vi "System Explorer - Copy Templates for System Explorer.vi"(7 "CD Name":string, 8 "error in (no error)":errorcluster, 10 "CD Template":refnum<class "NIVS_CD Template.lvclass">, 11 "System Explorer folder":path) -> (0 "error out":errorcluster)   [LabVIEW 2020, in "NIVS_Consolidated_CDW_MetaDataObj.lvclass"]
doc: "Copy the templates for the System Explorer library into the System Explorer folder and disconnect the templates from the owning library."
uses:
  NIVS_Consolidated_CDW_MetaDataObj.lvclass
  Template Classes/NIVS_CD Template/NIVS_CD Template.lvclass
  CD System Explorer lvlib.ctl
  Common.ctl
  CD Shared lvlib.ctl
  CD System Explorer lvlib.vi
  Common.vi
  CD Shared lvlib.vi
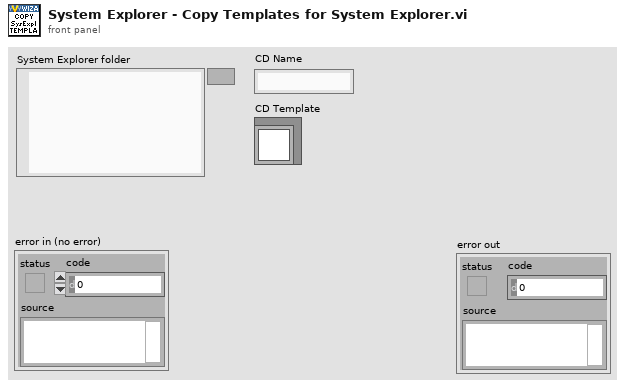
[diagram p1: front panel]
types:
  T1 = typedef "NIVS_Consolidated_CDW_MetaDataObj.lvclass/CD Shared lvlib.ctl" = enum16{"LibraryFileName", "LibraryFolderName", "ConstantsVI.VIPathAndName", "Shared.FolderName", "Shared.Types.FolderName", "Shared.Constants.VIName", "Shared.Constants.VITemplateName", "Shared.Constants.VITemplatePathAndName", "Shared.CompiledSettings.RelativePath", "Shared.Constants.RelativePath", "Shared.CompiledSettings.Name", "Shared.CompiledSettings.Name.NoExtension", "Shared.CompiledSettings.ClusterName"}
  T2 = typedef "NIVS_Consolidated_CDW_MetaDataObj.lvclass/CD System Explorer lvlib.ctl" = enum16{"LibraryFileName", "LibraryFolderName", "System Explorer.FolderName", "System Explorer.Dynamically Called.FolderName", "System Explorer.Dynamically Called.Extra Pages.FolderName", "System Explorer.Dynamically Called.Extra Pages.TemplatePathAndName", "System Explorer.Dynamically Called.Main Page.VIName", "System Explorer.Dynamically Called.Main Page.TemplatePathAndName", "System Explorer.Dynamically Called.Initialization VI.VIName", "System Explorer.Dynamically Called.Initialization VI.TemplatePathAndName", "System Explorer.SubVI.FolderName", "System Explorer.Types.FolderName", "System Explorer.ActionVIOnCompile.VIName", "System Explorer.ExportConfigRTM.VIName", "System Explorer.PPL.ExportConfigRTM.VIName", "System Explorer.LoadHelpFile.VIName", "System Explorer.PPL.LoadHelpFile.VIName", "System Explorer.SetRTDriverVIsFilePaths.VIName", "System Explorer.ClearRTDriverVIs.VIName"}
  T3 = typedef "NIVS_Consolidated_CDW_MetaDataObj.lvclass/Common.ctl" = enum16{"ProjectName", "TemplatesFolderName", "PPLTemplatesFolderName", "ProjectTemplatePathAndName", "ProjectPPLTemplatePathAndName", "TimingAndSyncFolderName", "CustomDeviceFolderName", "PathToTemplates", "PathToPPLTemplates", "PathToExplorerPPLTemplates", "PathToEnginePPLTemplates", "PathToConfigurationFile", "ProjectConfigurationName"}
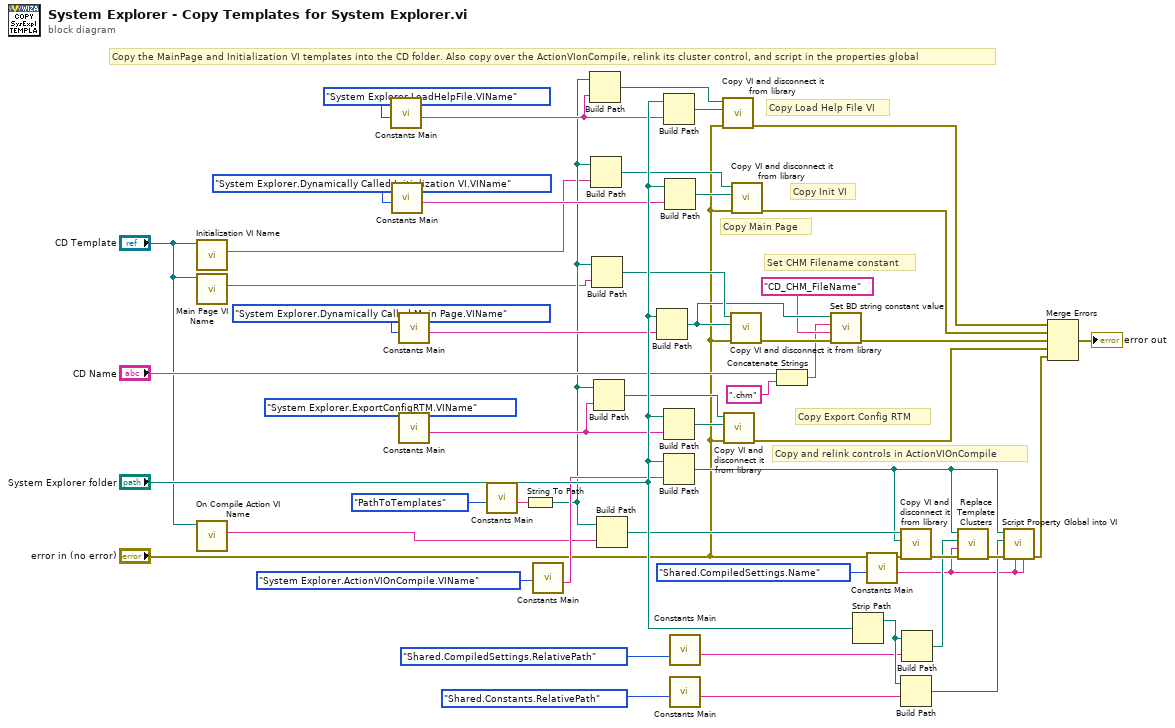
[diagram p0: block diagram]
diagram:
  # "Copy Load Help File VI"
  # "Copy the MainPage and Initialization VI templates into the CD folder. Also copy over the ActionVIonCompile, relink its cluster control, and script in the properties global"
  # "Set CHM Filename constant"
  # "Copy Export Config RTM"
  # "Copy and relink controls in ActionVIOnCompile"
  # "Copy Main Page"
  # "Copy Init VI"
  n1 = call-dynamic "Initialization VI Name.vi"("CD Template in"="CD Template") -> ("Initialization VI Name"=w6:string)  [unwired: 10 in]
  n2 = call-dynamic "Main Page VI Name.vi"("CD Template in"="CD Template") -> ("Main Page VI Name"=w5:string)  [unwired: 10 in]
  n3 = call-dynamic "On Compile Action VI Name.vi"("CD Template in"="CD Template") -> ("On Compile Action VI Name"=w4:string)  [unwired: 10 in]
  n4 = call-poly "Constants Main.vi"("Action"=CD_System_Explorer_lvlib."System Explorer.LoadHelpFile.VIName") -> ("Output"=w13:string)  [unwired: 10 in]
  n5 = call-poly "Constants Main.vi"("Action"=CD_System_Explorer_lvlib."System Explorer.Dynamically Called.Initialization VI.VIName") -> ("Output"=w39:string)  [unwired: 10 in]
  n6 = call-poly "Constants Main.vi"("Action"=CD_System_Explorer_lvlib."System Explorer.Dynamically Called.Main Page.VIName") -> ("Output"=w38:string)  [unwired: 10 in]
  n7 = call-poly "Constants Main.vi"("Action"=CD_System_Explorer_lvlib."System Explorer.ExportConfigRTM.VIName") -> ("Output"=w23:string)  [unwired: 10 in]
  n8 = call-poly "Constants Main.vi"("Action"=Common."PathToTemplates") -> ("Output"=w44:string)  [unwired: 10 in]
  n9 = String To Path(string=w44) -> (path=w9:path)
  n10 = call-poly "Constants Main.vi"("Action"=CD_System_Explorer_lvlib."System Explorer.ActionVIOnCompile.VIName") -> ("Output"=w31:string)  [unwired: 10 in]
  n11 = Build Path(base path=w9, name or relative path=w13) -> (appended path=w12:path)
  n12 = Build Path(base path=w9, name or relative path=w6) -> (appended path=w40:path)
  n13 = Build Path(base path=w9, name or relative path=w5) -> (appended path=w41:path)
  n14 = Build Path(base path=w9, name or relative path=w23) -> (appended path=w26:path)
  n15 = Build Path(base path=w9, name or relative path=w4) -> (appended path=w43:path)
  n16 = Build Path(base path="System Explorer folder", name or relative path=w38) -> (appended path=w19:path)
  n17 = Build Path(base path="System Explorer folder", name or relative path=w13) -> (appended path=w11:path)
  n18 = Build Path(base path="System Explorer folder", name or relative path=w23) -> (appended path=w25:path)
  n19 = Build Path(base path="System Explorer folder", name or relative path=w31) -> (appended path=w36:path)
  n20 = Build Path(base path="System Explorer folder", name or relative path=w39) -> (appended path=w47:path)
  n21 = call-poly "Constants Main.vi"("Action"=CD_Shared_lvlib."Shared.CompiledSettings.RelativePath") -> ("Output"=w1:string)  [unwired: 10 in]
  n22 = call-poly "Constants Main.vi"("Action"=CD_Shared_lvlib."Shared.Constants.RelativePath") -> ("Output"=w29:string)  [unwired: 10 in]
  n23 = call "Copy VI and disconnect it from library.vi"("error in (no error)"="error in (no error)", "VI Target Path"=w11, "VI Source Path"=w12) -> ("error out"=w8:errorcluster)  [unwired: 8 in]
  n24 = call "Copy VI and disconnect it from library.vi"("error in (no error)"="error in (no error)", "VI Target Path"=w25, "VI Source Path"=w26) -> ("error out"=w21:errorcluster)  [unwired: 8 in]
  n25 = call "Copy VI and disconnect it from library.vi"("error in (no error)"="error in (no error)", "VI Target Path"=w19, "VI Source Path"=w41) -> ("error out"=w20:errorcluster)  [unwired: 8 in]
  n26 = call "Copy VI and disconnect it from library.vi"("error in (no error)"="error in (no error)", "VI Target Path"=w47, "VI Source Path"=w40) -> ("error out"=w46:errorcluster)  [unwired: 8 in]
  n27 = Concatenate Strings("CD Name", ".chm" ("string")) -> (w15:string)
  n28 = call "Set BD string constant value.vi"("error in (no error)"=w20, "Name of string constant"="CD_CHM_FileName", "New String Value"=w15, "Path to VI"=w19) -> ("error out"=w17:errorcluster)  [unwired: 7 in]
  n29 = Strip Path(path="System Explorer folder") -> (stripped path=w34:path)  [unwired: 1 out]
  n30 = call-poly "Constants Main.vi"("Action"=CD_Shared_lvlib."Shared.CompiledSettings.Name") -> ("Output"=w28:string)  [unwired: 10 in]
  n31 = call "Copy VI and disconnect it from library.vi"("error in (no error)"="error in (no error)", "VI Target Path"=w36, "VI Source Path"=w43) -> ("error out"=w42:errorcluster)  [unwired: 8 in]
  n32 = Build Path(base path=w34, name or relative path=w29) -> (appended path=w33:path)
  n33 = Build Path(base path=w34, name or relative path=w1) -> (appended path=w35:path)
  n34 = call "Replace Template Clusters.vi"("error in (no error)"=w42, "Control Name"=w28, "Path to Cluster to Replace"=w35, "Path to VI"=w36) -> ("error out"=w37:errorcluster)  [unwired: 7 in]
  n35 = call "Script Property Global into VI.vi"("GlobalControlName"=w28, "StringConstantToReplace"=w28, "error in (no error)"=w37, "Path to Global"=w33, "Path to VI"=w36) -> ("error out"=w22:errorcluster)  [unwired: 6 in]
  n36 = Merge Errors(w8, w46, w17, w21, w22) -> (→"error out":errorcluster)
